vi "testMaxMin.vi"(5 "valesAmplitude in":dbl[](array[numeric]), 6 "peaksAmplitude in":dbl[](array[numeric]), 7 "Error In":errorcluster, 8 "iPeaksLocation in":dbl[](array[numeric]), 9 "iValesLocation in":dbl[](array[numeric]), 10 "passThreshold":i32[](array[numeric])) -> (0 "Error Out":errorcluster, 1 "iValesLocation out":dbl[](array[numeric]), 2 "peaksAmplitude out":dbl[](array[numeric]), 3 "iPeaksLocation out":dbl[](array[numeric]), 4 "valesAmplitude out":dbl[](array[numeric]))   [LabVIEW 2015]
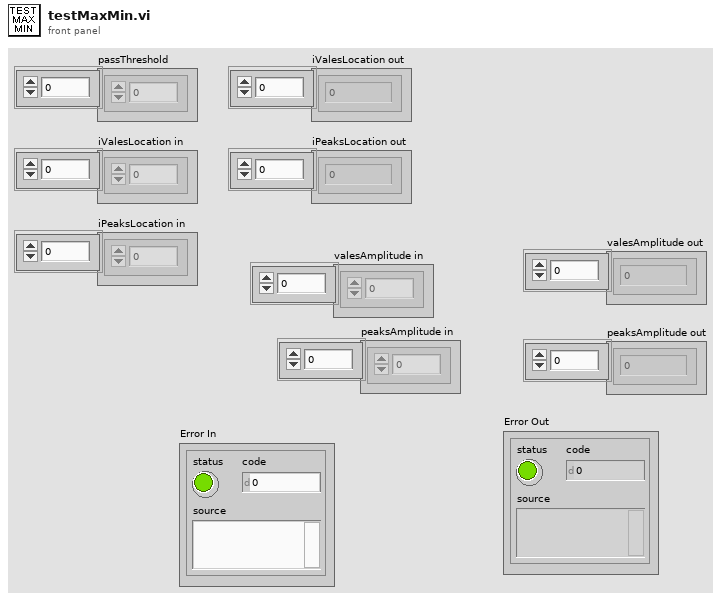
[diagram p1: front panel]
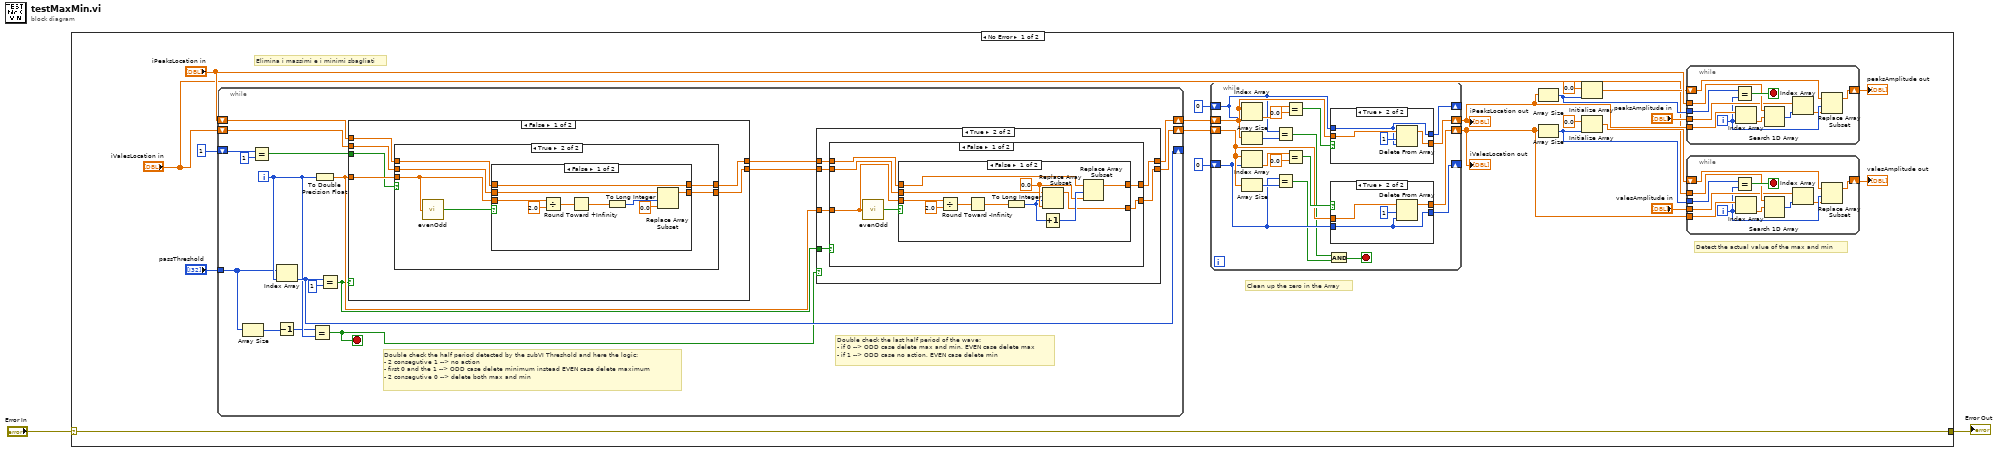
[diagram p0: block diagram]
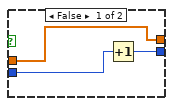
[diagram p2: hidden frame]
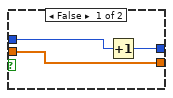
[diagram p3: hidden frame]
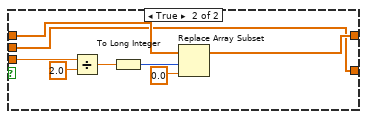
[diagram p5: hidden frame]
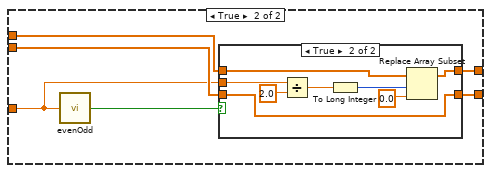
[diagram p6: hidden frame]
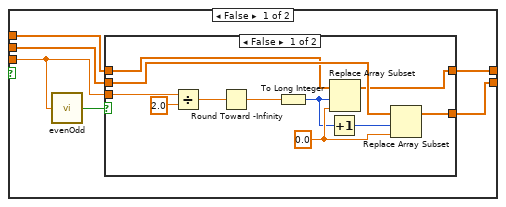
[diagram p8: hidden frame]
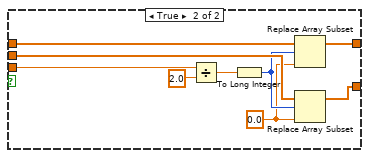
[diagram p9: hidden frame]
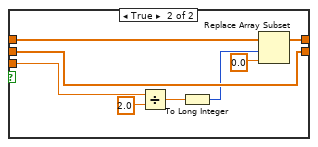
[diagram p10: hidden frame]
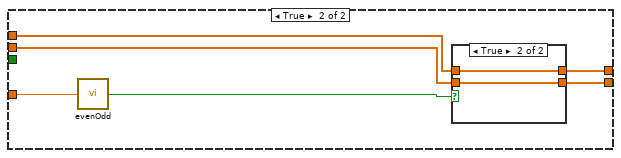
[diagram p11: hidden frame]
diagram:
  n1 = case shown="No Error" "Error In" {
    selector: "Error In" -> [w3 w211]
    tunnel: [w3 w211] -> w1
    frame No Error {
      # "Detect the actual value of the max and min"
      # "Clean up the zero in the Array"
      # "Elimina i massimi e i minimi sbagliati"
      n2 = while {
        tunnel: "passThreshold" -> [w80]
        shift-right: [w83] -> w20
        shift-left: "iPeaksLocation in" -> [w95]
        shift-right: [w84] -> w21
        shift-left: "iValesLocation in" -> [w94]
        shift-right: [w93] -> _
        shift-left: 1 ("element") -> [w92]
        i -> [w89]
        stop <- w85 stop-if-true
        # "Double check the last half period of the wave:\n- if 0 --> ODD case delete max and min, EVEN case delete max\n- if 1 --> ODD case no action, EVEN case delete min"
        # "Double check the half period detected by the subVI Threshold and here the logic:\n- 2 consegutive 1 --> no action\n- first 0 and the 1 --> ODD case delete minimum instead EVEN case delete maximum\n- 2 consegutive 0 --> delete both max and min"
        n3 = Array Size(array=w80) -> (size(s)=w88:i32)
        n4 = Equal?(x=w92, y=1) -> (x = y?=w90:bool)
        n5 = Decrement(x=w88) -> (x-1=w82:i32)
        n6 = Index Array(array=w80, index=w89) -> (element=w93:i32)
        n7 = Equal?(x=w82, y=w89) -> (x = y?=w85:bool)
        n8 = To Double Precision Float(number=w89) -> (double precision float=w81:dbl)
        n9 = Equal?(x=w93, y=1) -> (x = y?=w79:bool)
        n10 = case shown="False" w79 {
          tunnel: w81 -> [w151 w206]
          tunnel: w95 -> [w150 w204]
          tunnel: w94 -> [w149 w202]
          tunnel: [w148 w203] -> w86
          tunnel: [w147 w201] -> w87
          tunnel: w90 -> [w146 _]
          frame False {
            n11 = case shown="True" w146 {
              tunnel: w151 -> [w152 w178]
              tunnel: w150 -> [w155 w182]
              tunnel: w149 -> [w157 w179]
              tunnel: [w154 w181] -> w148
              tunnel: [w156 w180] -> w147
              frame False {
                n12 = call "evenOdd.vi"("number"=w152) -> ("odd/even"=w153:bool)
                n13 = case shown="False" w153 {
                  tunnel: w157 -> [w168 w177]
                  tunnel: [w167 w176] -> w156
                  tunnel: w155 -> [w158 w175]
                  tunnel: [w166 w174] -> w154
                  tunnel: w152 -> [w165 w173]
                  frame False {
                    w161 = 0.0 ("new element/subarray")
                    n14 = Divide(x=w165, y=2.0) -> (x/y=w163:dbl)
                    n15 = Round Toward -Infinity(1:w163) -> (0:w162:dbl)
                    n16 = To Long Integer(number=w162) -> (32bit integer=w160:i32)
                    n17 = Increment(x=w160) -> (x+1=w159:i32)
                    n18 = Replace Array Subset(array=w158, new element=w161, index=w160) -> (w166:dbl[])
                    n19 = Replace Array Subset(array=w168, new element=w161, index=w159) -> (w167:dbl[])
                  }
                  frame True {
                    w169 = 0.0 ("new element/subarray")
                    n20 = Divide(x=w173, y=2.0) -> (x/y=w171:dbl)
                    n21 = To Long Integer(number=w171) -> (32bit integer=w170:i32)
                    n22 = Replace Array Subset(array=w175, new element=w169, index=w170) -> (w174:dbl[])
                    n23 = Replace Array Subset(array=w177, new element=w169, index=w170) -> (w176:dbl[])
                  }
                }
              }
              frame True {
                n24 = call "evenOdd.vi"("number"=w178) -> ("odd/even"=w183:bool)
                n25 = case shown="False" w183 {
                  tunnel: w182 -> [w190 w200]
                  tunnel: w179 -> [w192 w198]
                  tunnel: w178 -> [w188 w195]
                  tunnel: [w190 w199] -> w181
                  tunnel: [w191 w198] -> w180
                  frame False {
                    n26 = Divide(x=w188, y=2.0) -> (x/y=w186:dbl)
                    n27 = Round Toward +Infinity(x=w186) -> (ceil(x): smallest int >= x=w185:dbl)
                    n28 = To Long Integer(number=w185) -> (32bit integer=w184:i32)
                    n29 = Replace Array Subset(array=w192, new element=0.0 ("new element/subarray"), index=w184) -> (w191:dbl[])
                  }
                  frame True {
                    n30 = Divide(x=w195, y=2.0) -> (x/y=w193:dbl)
                    n31 = To Long Integer(number=w193) -> (32bit integer=w196:i32)
                    n32 = Replace Array Subset(array=w200, new element=0.0 ("length"), index=w196) -> (w199:dbl[])
                  }
                }
              }
            }
          }
          frame True {
            n33 = call "evenOdd.vi"("number"=w206) -> ("odd/even"=w205:bool)
            n34 = case shown="True" w205 {
              tunnel: w204 -> [w208 w210]
              tunnel: [w208 w210] -> w203
              tunnel: w202 -> [w207 w209]
              tunnel: [w207 w209] -> w201
              frame False {
              }
              frame True {
              }
            }
          }
        }
        n35 = case shown="True" w85 {
          tunnel: w87 -> [w98 w104]
          tunnel: w86 -> [w97 w101]
          tunnel: w81 -> [_ w103]
          tunnel: [w98 w102] -> w84
          tunnel: [w97 w100] -> w83
          tunnel: w79 -> [_ w99]
          frame False {
          }
          frame True {
            n36 = case shown="False" w99 {
              tunnel: w104 -> [w109 w134]
              tunnel: w103 -> [w105 w133]
              tunnel: [w107 w132] -> w102
              tunnel: w101 -> [w108 w131]
              tunnel: [w106 w130] -> w100
              frame False {
                n37 = call "evenOdd.vi"("number"=w105) -> ("odd/even"=w110:bool)
                n38 = case shown="False" w110 {
                  tunnel: w109 -> [w115 w127]
                  tunnel: w108 -> [w114 w129]
                  tunnel: [w113 w127] -> w107
                  tunnel: [w112 w128] -> w106
                  tunnel: w105 -> [w111 w126]
                  frame False {
                    w120 = 0.0 ("new element/subarray")
                    n39 = Divide(x=w111, y=2.0) -> (x/y=w117:dbl)
                    n40 = Round Toward -Infinity(1:w117) -> (0:w118:dbl)
                    n41 = To Long Integer(number=w118) -> (32bit integer=w119:i32)
                    n42 = Increment(x=w119) -> (x+1=w121:i32)
                    n43 = Replace Array Subset(array=w115, new element=w120, index=w119) -> (w113:dbl[])
                    n44 = Replace Array Subset(array=w114, new element=w120, index=w121) -> (w112:dbl[])
                  }
                  frame True {
                    n45 = Divide(x=w126, y=2.0) -> (x/y=w124:dbl)
                    n46 = To Long Integer(number=w124) -> (32bit integer=w123:i32)
                    n47 = Replace Array Subset(array=w129, new element=0.0 ("new element/subarray"), index=w123) -> (w128:dbl[])
                  }
                }
              }
              frame True {
                n48 = call "evenOdd.vi"("number"=w133) -> ("odd/even"=w135:bool)
                n49 = case shown="True" w135 {
                  tunnel: w134 -> [w136 w138]
                  tunnel: w133 -> [_ w145]
                  tunnel: [w136 w138] -> w132
                  tunnel: w131 -> [w137 w140]
                  tunnel: [w137 w139] -> w130
                  frame False {
                  }
                  frame True {
                    n50 = Divide(x=w145, y=2.0) -> (x/y=w143:dbl)
                    n51 = To Long Integer(number=w143) -> (32bit integer=w142:i32)
                    n52 = Replace Array Subset(array=w140, new element=0.0 ("new element/subarray"), index=w142) -> (w139:dbl[])
                  }
                }
              }
            }
          }
        }
      }
      n53 = while {
        shift-right: [w57] -> w15
        shift-left: w20 -> [w50]
        shift-right: [w58] -> w6
        shift-left: w21 -> [w54]
        shift-right: [w56] -> _
        shift-left: 0 -> [w52]
        shift-right: [w55] -> _
        shift-left: 0 -> [w46]
        stop <- w47 stop-if-true
        n54 = Index Array(array=w50, index=w46) -> (element=w64:dbl)
        n55 = Array Size(array=w50) -> (size(s)=w51:i32)
        n56 = Index Array(array=w54, index=w52) -> (element=w61:dbl)
        n57 = Array Size(array=w54) -> (size(s)=w53:i32)
        n58 = Equal?(x=w46, y=w51) -> (x = y?=w48:bool)
        n59 = Equal?(x=w52, y=w53) -> (x = y?=w49:bool)
        n60 = Equal?(x=w64, y=0.0) -> (x = y?=w62:bool)
        n61 = Equal?(x=w61, y=0.0) -> (x = y?=w59:bool)
        n62 = And(x=w48, y=w49) -> (x .and. y?=w47:bool)
        n63 = case shown="True" w62 {
          tunnel: w50 -> [w72 w78]
          tunnel: [w72 w77] -> w57
          tunnel: [w74 w75] -> w55
          tunnel: w46 -> [w73 w75]
          frame False {
            n64 = Increment(x=w73) -> (x+1=w74:i32)
          }
          frame True {
            n65 = Delete From Array(array=w78, length=1, index=w75) -> (array with subset deleted=w77:dbl[])  [unwired: 1 out]
          }
        }
        n66 = case shown="True" w59 {
          tunnel: w54 -> [w65 w71]
          tunnel: [w65 w70] -> w58
          tunnel: [w67 w68] -> w56
          tunnel: w52 -> [w66 w68]
          frame False {
            n67 = Increment(x=w66) -> (x+1=w67:i32)
          }
          frame True {
            n68 = Delete From Array(array=w71, length=1, index=w68) -> (array with subset deleted=w70:dbl[])  [unwired: 1 out]
          }
        }
      }
      "iPeaksLocation out" <- w15
      "iValesLocation out" <- w6
      n69 = Array Size(array=w15) -> (size(s)=w14:i32)
      n70 = Array Size(array=w6) -> (size(s)=w10:i32)
      n71 = Initialize Array(0.0 ("element"), w14) -> (w12:dbl[])
      n72 = Initialize Array(0.0 ("element"), w10) -> (w8:dbl[])
      n73 = while {
        tunnel: "iPeaksLocation in" -> [w42]
        tunnel: w15 -> [w44]
        tunnel: "peaksAmplitude in" -> [w40]
        tunnel: w14 -> [w41]
        shift-right: [w37] -> w11
        shift-left: w12 -> [w38]
        i -> [w36]
        stop <- w45 stop-if-true
        n74 = Equal?(x=w41, y=w36) -> (x = y?=w45:bool)
        n75 = Index Array(array=w44, index=w36) -> (element=w43:dbl)
        n76 = Search 1D Array(1D array=w42, element=w43) -> (index of element=w39:i32)  [unwired: 1 in]
        n77 = Index Array(array=w40, index=w39) -> (element=w35:dbl)
        n78 = Replace Array Subset(array=w38, new element=w35, index=w36) -> (w37:dbl[])
      }
      "peaksAmplitude out" <- w11
      n79 = while {
        tunnel: "iValesLocation in" -> [w31]
        tunnel: w6 -> [w33]
        tunnel: "valesAmplitude in" -> [w29]
        tunnel: w10 -> [w30]
        shift-right: [w26] -> w4
        shift-left: w8 -> [w27]
        i -> [w25]
        stop <- w34 stop-if-true
        n80 = Equal?(x=w30, y=w25) -> (x = y?=w34:bool)
        n81 = Index Array(array=w33, index=w25) -> (element=w32:dbl)
        n82 = Search 1D Array(1D array=w31, element=w32) -> (index of element=w28:i32)  [unwired: 1 in]
        n83 = Index Array(array=w29, index=w28) -> (element=w24:dbl)
        n84 = Replace Array Subset(array=w27, new element=w24, index=w25) -> (w26:dbl[])
      }
      "valesAmplitude out" <- w4
    }
    frame Error {
    }
  }
  "Error Out" <- w1
